vi "DB_Migration.vi"() -> ()   [LabVIEW 2020]
uses:
  <vilib>/addons/database/Connection.llb/DB Tools Open Connec (String).vi
  <vilib>/addons/database/NI_Database_API.lvlib
panel:
  out "error out":errorcluster
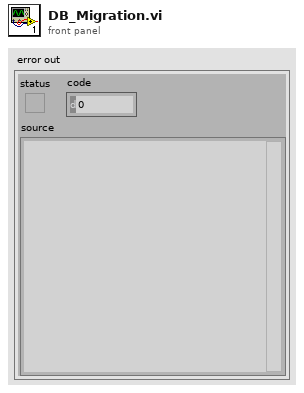
[diagram p1: front panel]
types:
  T1 = enum32{"invalid app kind", "Development System", "Run Time System", "Student Edition", "Embedded LabVIEW", "Evaluation", "Custom"}
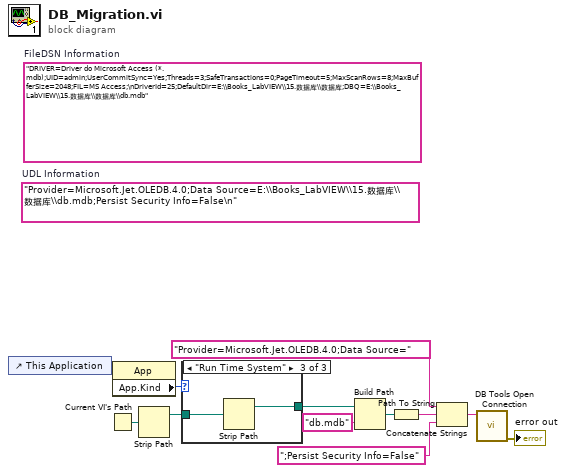
[diagram p0: block diagram]
diagram:
  (unwired) "Provider=Microsoft.Jet.OLEDB.4.0;Data Source=E:\\Books_LabVIEW\\15.数据库\\数据库\\db.mdb;Persist Security Info=False\n"  # UDL Information
  (unwired) "DRIVER=Driver do Microsoft Access (*.mdb);UID=admin;UserCommitSync=Yes;Threads=3;SafeTransactions=0;PageTimeout=5;MaxScanRows=8;MaxBufferSize=2048;FIL=MS Access;\nDriverId=25;DefaultDir=E:\\Books_LabVIEW\\15.数据库\\数据库;DBQ=E:\\Books_LabVIEW\\15.数据库\\数据库\\db.mdb"  # FileDSN Information
  n1 = control-ref of="This Application"() -> (w5:refnum<vi>)
  n2 = Current VI's Path() -> (path=w6:path)
  n3 = property class="App"(reference=w5) -> ("App.Kind"=w4:T1)  [unwired: 1 in, 2 out]
  n4 = Strip Path(path=w6) -> (stripped path=w3:path)  [unwired: 1 out]
  n5 = case shown="\"Run Time System\"" w4 {
    tunnel: w3 -> [w13 w14 w16]
    tunnel: [w13 w14 w15] -> w2
    frame "invalid app kind", Default {
    }
    frame "Development System" {
    }
    frame "Run Time System" {
      n6 = Strip Path(path=w16) -> (stripped path=w15:path)  [unwired: 1 out]
    }
  }
  n7 = Build Path(base path=w2, name or relative path="db.mdb" ("Filename")) -> (appended path=w10:path)
  n8 = Path To String(path=w10) -> (string=w9:string)
  n9 = Concatenate Strings("Provider=Microsoft.Jet.OLEDB.4.0;Data Source=" ("string"), w9, ";Persist Security Info=False" ("string")) -> (w1:string)
  n10 = call-poly <vilib>:"DB Tools Open Connection.vi"("connection information"=w1) -> ("error out"=→"error out":errorcluster)  [unwired: 7 in, 1 out]
